vi "AccCmdGenerate.vi"(1 "Acceleration":sgl=1.5 format="%.4f", 3 "Dst":i32=54 format="%x") -> (0 "CMD code":string)   [LabVIEW 2012]
panel:
  out "Revised":u8[](array[numeric]) format="%02x"
  out "Array":u8[](array[numeric]) format="%02x"
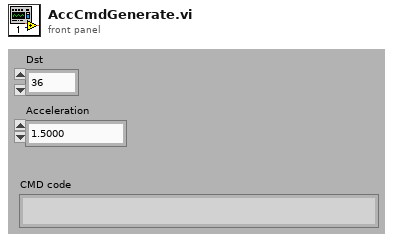
[diagram p1: front panel]
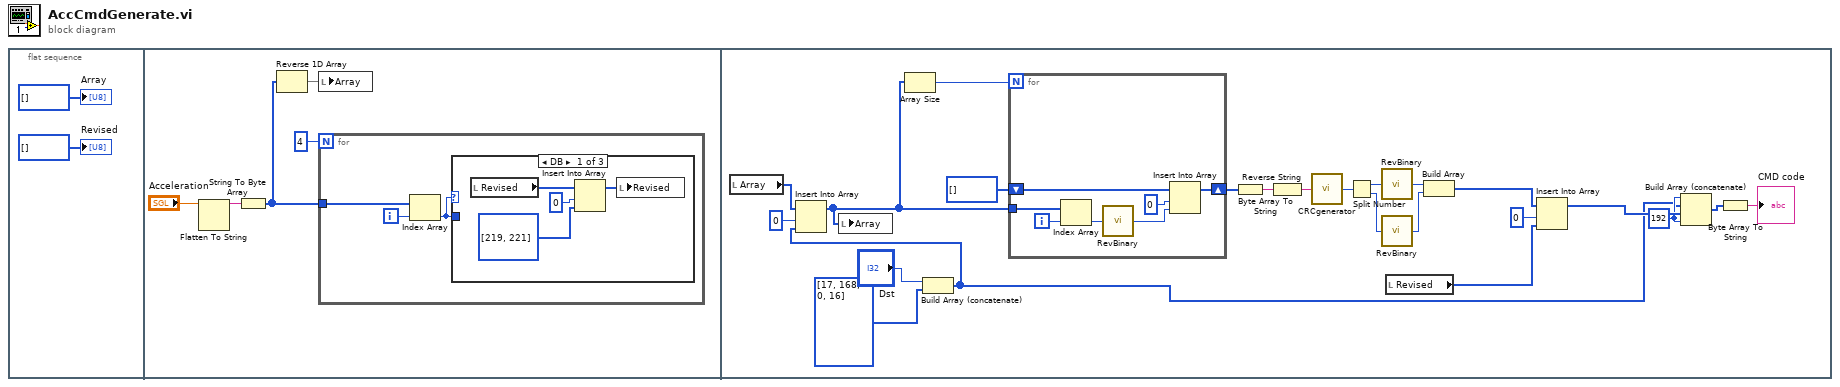
[diagram p0: block diagram]
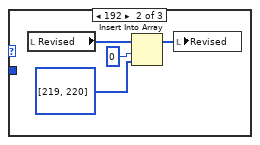
[diagram p2: hidden frame]
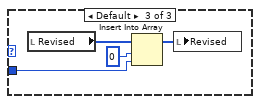
[diagram p3: hidden frame]
diagram:
  n1 = flat-sequence {
    frame #0 {
      "Array" <- u8[] []
      "Revised" <- u8[] []
    }
    frame #1 {
      n2 = Flatten To String(anything="Acceleration") -> (data string=w6:string)  [unwired: 3 in, 2 out]
      n3 = String To Byte Array(string=w6) -> (unsigned byte array=w4:u8[])
      n4 = Reverse 1D Array(array=w4) -> (reversed array=w3:u8[])
      n5 = local write "Array"(w3) -> ()
      n6 = for {
        N: 4 -> [_]
        tunnel: w4 -> [w9]
        i -> [w10]
        n7 = Index Array(array=w9, index=w10) -> (element=w8:u8)
        n8 = case shown="DB" w8 {
          tunnel: w8 -> [_ _ w22]
          frame 219 {
            n9 = local read "Revised"() -> (w11:u8[])
            n10 = Insert Into Array(array=w11, index=0, new element=i32[] [219, 221]) -> (w13:u8[])
            n11 = local write "Revised"(w13) -> ()
          }
          frame 192 {
            n12 = local read "Revised"() -> (w16:u8[])
            n13 = Insert Into Array(array=w16, index=0, new element=i32[] [219, 220]) -> (w15:u8[])
            n14 = local write "Revised"(w15) -> ()
          }
          frame Default {
            n15 = local read "Revised"() -> (w19:u8[])
            n16 = Insert Into Array(array=w19, index=0, new element=w22) -> (w21:u8[])
            n17 = local write "Revised"(w21) -> ()
          }
        }
      }
    }
    frame #2 {
      w24 = 192
      n18 = local read "Array"() -> (w45:u8[])
      n19 = Build Array (concatenate)("Dst", i32[] [17, 168, 0, 16]) -> (w23:i32[])
      n20 = Insert Into Array(array=w45, index=0, new element=w23) -> (w42:u8[])
      n21 = local write "Array"(w42) -> ()
      n22 = Array Size(array=w42) -> (size(s)=w43:i32)
      n23 = for {
        N: w43 -> [_]
        tunnel: w42 -> [w52]
        shift-right: [w49] -> w38
        shift-left: u32[] [] -> [w48]
        i -> [w51]
        n24 = Index Array(array=w52, index=w51) -> (element=w47:u8)
        n25 = call "RevBinary.vi"("Binary"=w47) -> ("Rev Binary"=w46:u32)
        n26 = Insert Into Array(array=w48, index=0, new element=w46) -> (w49:u32[])
      }
      n27 = Byte Array To String(unsigned byte array=w38) -> (string=w39:string)
      n28 = Reverse String(1:w39) -> (0:w40:string)
      n29 = call "CRCgenerator.vi"("String"=w40) -> ("CRC-16-CCITT-0xFFFF"=w37:u16)
      n30 = Split Number(x=w37) -> (hi(x)=w36:u8, lo(x)=w35:u8)
      n31 = call "RevBinary.vi"("Binary"=w36) -> ("Rev Binary"=w32:u32)
      n32 = call "RevBinary.vi"("Binary"=w35) -> ("Rev Binary"=w31:u32)
      n33 = local read "Revised"() -> (w33:u8[])
      n34 = Build Array(w32, w31) -> (w30:u32[])
      n35 = Insert Into Array(array=w30, index=0, new element=w33) -> (w27:u32[])
      n36 = Build Array (concatenate)(w24, w23, w27, w24) -> (w29:u32[])
      n37 = Byte Array To String(unsigned byte array=w29) -> (string=→"CMD code":string)
    }
  }
